vi "CleanUp.vi"(0 "Process In":refnum<class "Process.lvclass">, 1 "Timeout in ms (-1)":i32=-1, 11 "Error In":errorcluster) -> (4 "Process Out":refnum<class "Process.lvclass">, 15 "Error Out":errorcluster)   [LabVIEW 2023, in "Process.lvclass"]
uses:
  Process.lvclass
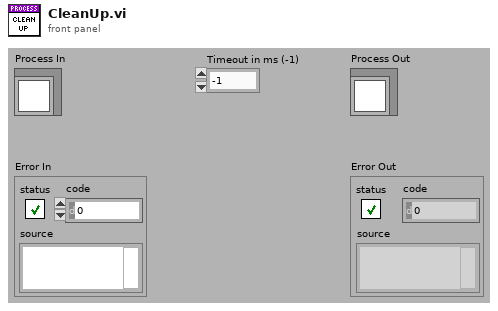
[diagram p1: front panel]
types:
  T1 = enum16{"ReadRepository", "CreateNew", "CreateOrLookUpExisting", "ReadRepositoryAndDestroy"}
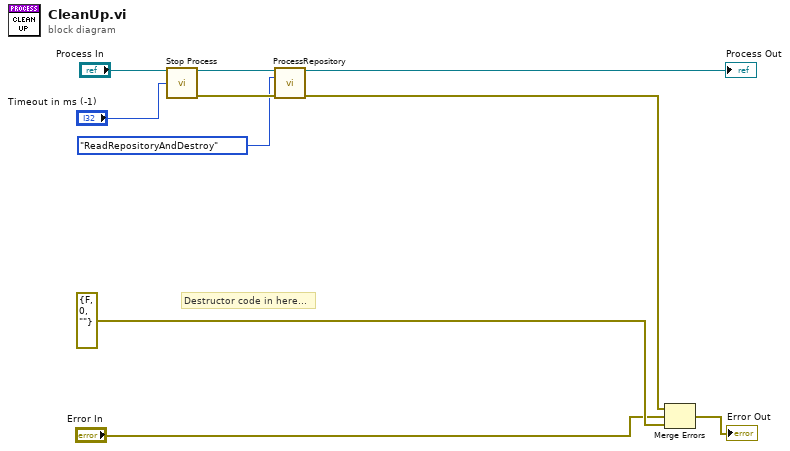
[diagram p0: block diagram]
diagram:
  # "Destructor code in here..."
  n1 = call-dynamic "Stop Process.vi"("Process In"="Process In", "ms Timeout (-1)"="Timeout in ms (-1)") -> ("Process Out"=w3:refnum<class "Process.lvclass">, "Error Out"=w6:errorcluster)  [unwired: 12 in]
  n2 = call-dynamic "ProcessRepository.vi"("Process In"=w3, "Action(ReadRepository)"=T1."ReadRepositoryAndDestroy", "Error In"=w6) -> ("Process Out"=→"Process Out":refnum<class "Process.lvclass">, "Error Out"=w4:errorcluster)  [unwired: 6 in, 5 out]
  n3 = Merge Errors(w4, "Error In", errorcluster {"status"=FALSE, "code"=0, "source"=""} ("error in (no error)")) -> (→"Error Out":errorcluster)
